vi "TTA_Format_IP_Address_Into_VISA.vi"(8 "error in":errorcluster, 11 "IP Address":string) -> (0 "error out":errorcluster, 3 "VISA resource name":refnum<visa-resource-name>)   [LabVIEW 2016]
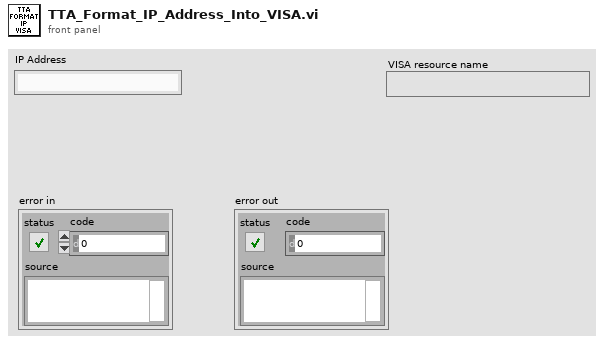
[diagram p1: front panel]
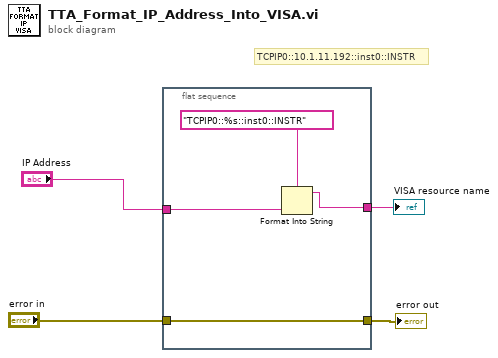
[diagram p0: block diagram]
diagram:
  # "TCPIP0::10.1.11.192::inst0::INSTR"
  n1 = flat-sequence {
    tunnel: "IP Address" -> [w6]
    tunnel: "error in" -> [w8]
    tunnel: [w8] -> w2
    tunnel: [w5] -> w1
    frame #0 {
      n2 = Format Into String(format string="TCPIP0::%s::inst0::INSTR", w6) -> (resulting string=w5:string)  [unwired: 2 in, 1 out]
    }
  }
  "error out" <- w2
  "VISA resource name" <- w1
